vi "Lengmure_s_probe2.vi"() -> ()   [LabVIEW 2013]
uses:
  <vilib>/Instr/_visa.llb/VISA Configure Serial Port (Instr).vi
  <vilib>/Utility/file.llb/Write To Spreadsheet File (DBL).vi
  convert.dll
panel:
  out "?":dynamicdata(graph)
  in  "Tab Control":T1(tab)
  in  "Start":bool
  out "Имя соединения":refnum<visa-resource-name>
  in  "Компорт":refnum<visa-resource-name>="COM4"
  in  "Скорость передачи":u32=9600
  in  "Токоограничитель":bool=TRUE
  in  "50 герцовый фильтр":bool
  in  "Опорное напряжение АЦП, Вольты":dbl=5.0
  in  "Разрядность АЦП":u8=10
  in  "Реле 4":bool
  in  "Реле 3":bool
  in  "Реле 2":bool
  in  "Реле 1":bool
  in  "Go":bool
  in  "Save":bool
  in  "Clear":bool
  in  "stop":bool
  out "U-I Diagram":cluster{dbl[], dbl[]}(graph)
  in  "Команда":string
  out "Отправка команд /Чтение данных":bool
  in  "Начальное напряжение(0..255)":u8
  in  "Диапазон напряжения(0..255)":u8=255
  in  "Задержка (10 мс)(0..255)":u8=1
  in  "Количество шагов(0..255)":u8=255
  in  "Повторы(0..255)":u8=1
  in  "Время паузы данных(мс)":u32=1000
  in  "Обратный коэффицент делителя напряжения, Безразм":dbl=49.0
  in  "Сопротивление шунта, Ом":dbl=22.0
  out "Время выполнения операции(мсек)":u32
  out "Передача команд":errorcluster
  out "Инициализация":errorcluster
  out "Модуль считывания данных":errorcluster
  out "Закрытие соединения":errorcluster
  out "Вспомогательная переменная времени начала команды":u32
  out "Вспомогательная переменная времени последних принятых данных":u32
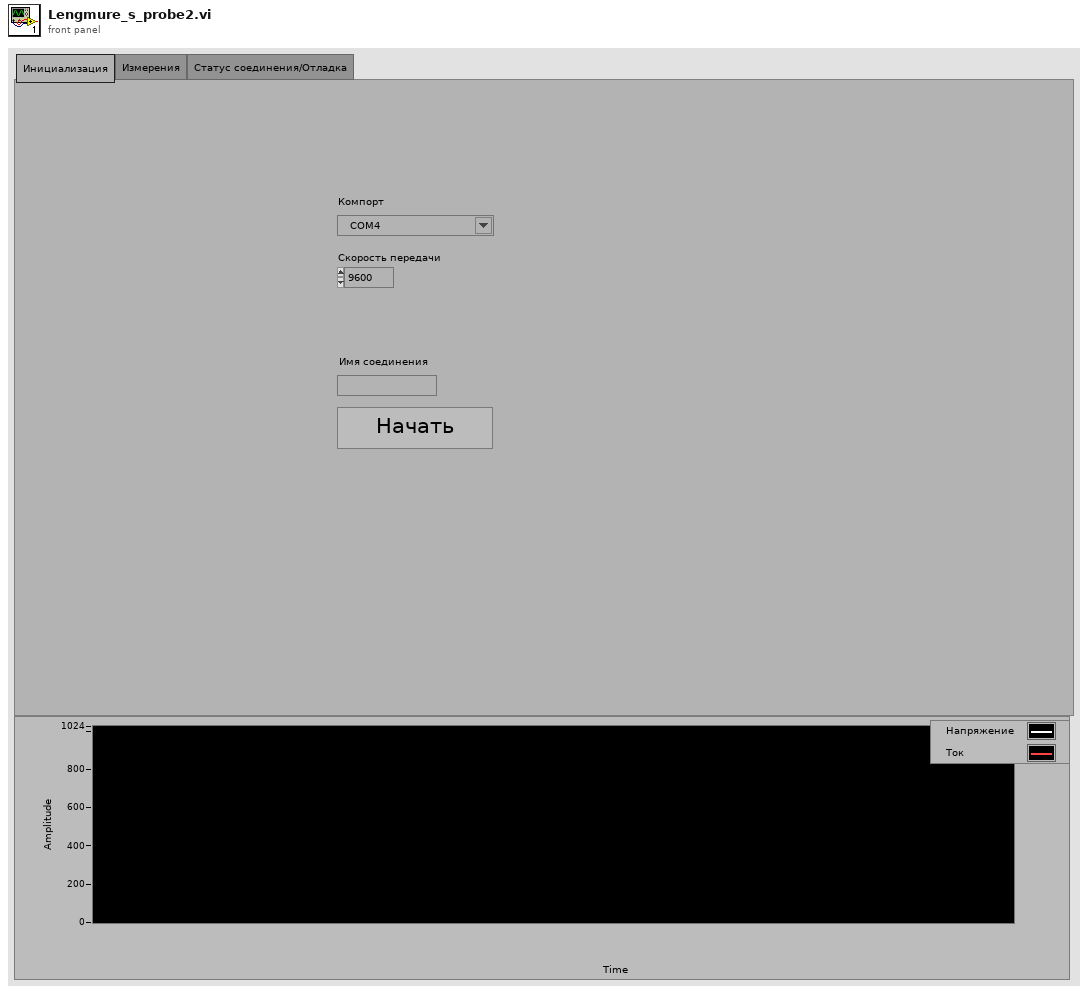
[diagram p1: front panel]
types:
  T1 = enum32{"Инициализация", "Измерения", "Статус соединения/Отладка"}
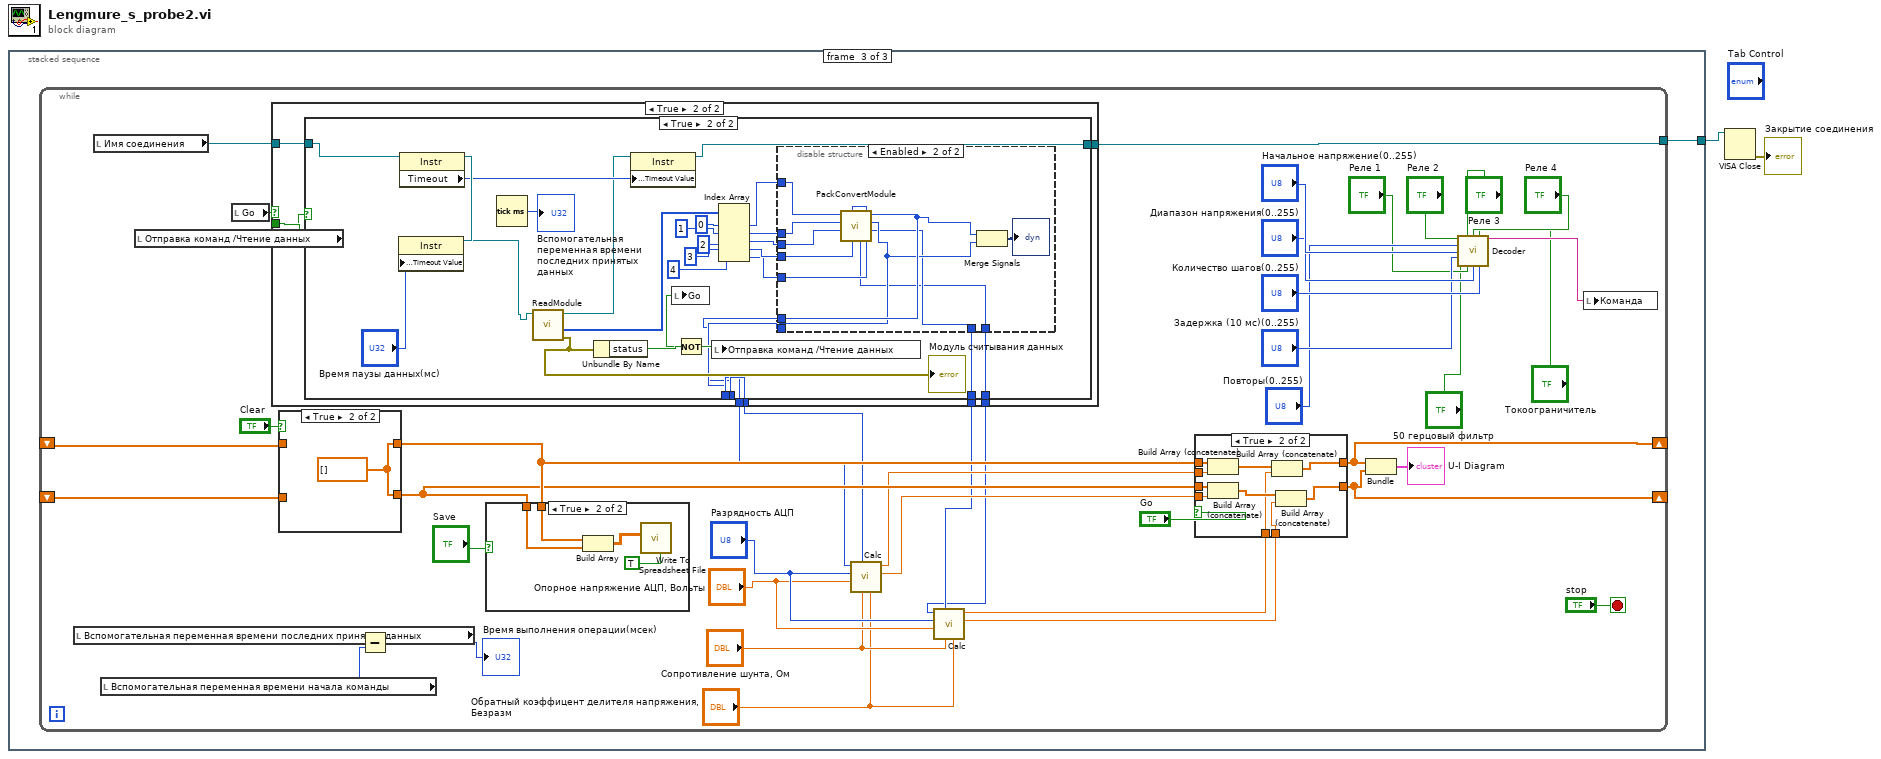
[diagram p0: block diagram]
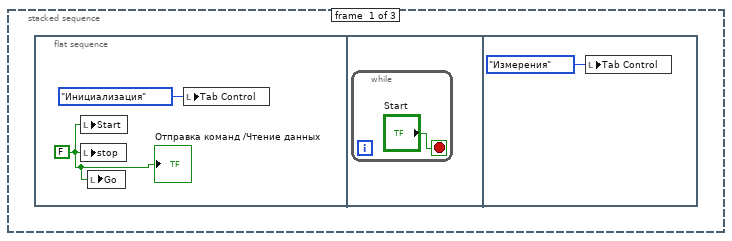
[diagram p2: hidden frame]
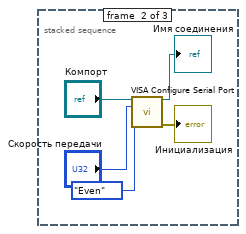
[diagram p3: hidden frame]
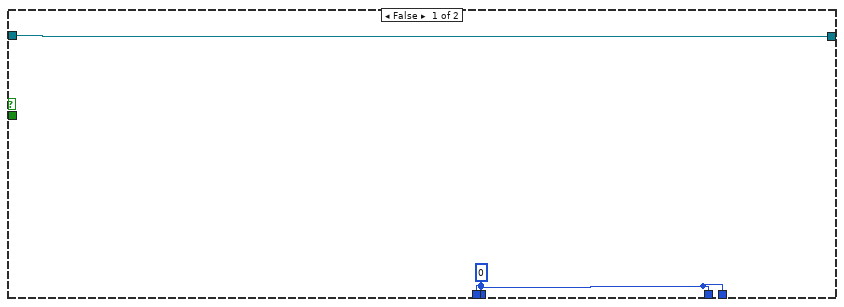
[diagram p4: hidden frame]
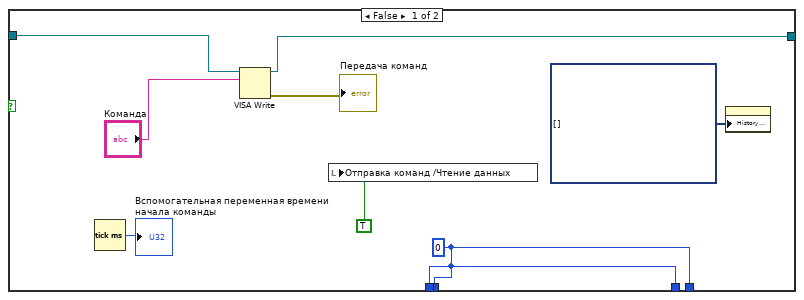
[diagram p5: hidden frame]
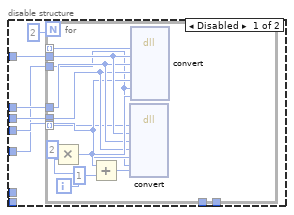
[diagram p6: hidden frame]
diagram:
  n1 = stacked-sequence {
    tunnel: [_ _ w12] -> w2
    frame #0 {
      n2 = flat-sequence {
        frame #0 {
          w3 = FALSE ("Start")
          n3 = local write "Start"(w3) -> ()
          n4 = local write "stop"(w3) -> ()
          n5 = local write "Go"(w3) -> ()
          n6 = local write "Tab Control"(enum32{"Инициализация", "Измерения"}."Инициализация" ("Tab Control")) -> ()
          "Отправка команд /Чтение данных" <- w3
        }
        frame #1 {
          n7 = while {
            stop <- "Start" stop-if-true
          }
        }
        frame #2 {
          n8 = local write "Tab Control"(enum32{"Инициализация", "Измерения"}."Измерения" ("Tab Control")) -> ()
        }
      }
    }
    frame #1 {
      n9 = call-poly "VISA Configure Serial Port"("VISA resource name"="Компорт", "baud rate (9600)"="Скорость передачи", "parity (0:none)"=enum16{"None", "Odd", "Even", "Mark", "Space"}."Even") -> ("VISA resource name out"=→"Имя соединения":refnum<visa-resource-name>, "error out"=→"Инициализация":errorcluster)  [unwired: 11 in]
    }
    frame #2 {
      n10 = while {
        shift-right: [w41] -> _
        shift-left: _ -> [w53]
        shift-right: [w40] -> _
        shift-left: _ -> [w52]
        tunnel: [w45] -> w12
        stop <- "stop" stop-if-true
        n11 = local read "Вспомогательная переменная времени последних принятых данных"() -> (w22:u32)
        n12 = local read "Имя соединения"() -> (w46:refnum<visa-resource-name>)
        n13 = local read "Вспомогательная переменная времени начала команды"() -> (w23:u32)
        n14 = local read "Отправка команд /Чтение данных"() -> (w43:bool)
        n15 = local read "Go"() -> (w44:bool)
        n16 = case shown="True" w44 {
          tunnel: [w55 w63] -> w27
          tunnel: [w55 w62] -> w26
          tunnel: w46 -> [w56 w61]
          tunnel: [w56 w60] -> w45
          tunnel: w43 -> [_ w59]
          tunnel: [w55 w58] -> w20
          tunnel: [w55 w57] -> w19
          frame False {
            w55 = u16 0 ("return type")
          }
          frame True {
            n17 = case shown="True" w59 {
              tunnel: [w64 w75] -> w63
              tunnel: [w64 w76] -> w62
              tunnel: w61 -> [w71 w93]
              tunnel: [w70 w92] -> w60
              tunnel: [w64 w73] -> w58
              tunnel: [w64 w72] -> w57
              frame False {
                w64 = 0
                n18 = Tick Count (ms)() -> (millisecond timer value=→"Вспомогательная переменная времени начала команды":u32)
                n19 = VISA Write(VISA resource name=w71, write buffer="Команда") -> (VISA resource name out=w70:refnum<visa-resource-name>, error out=→"Передача команд":errorcluster)  [unwired: 1 in, 1 out]
                n20 = local write "Отправка команд /Чтение данных"(TRUE) -> ()
                n21 = property class="WFChart (strict)"("History Data"=dynamicdata[] []) -> ()  [unwired: 2 in, 2 out]
              }
              frame True {
                n22 = property class="Instr"(reference=w93) -> (reference out=w94:refnum<visa-resource-name>, "Timeout"=w91:u32)  [unwired: 1 in, 1 out]
                n23 = property class="Instr"(reference=w94, "General Settings:Timeout Value"="Время паузы данных(мс)") -> (reference out=w80:refnum<visa-resource-name>)  [unwired: 1 in, 1 out]
                n24 = Tick Count (ms)() -> (millisecond timer value=→"Вспомогательная переменная времени последних принятых данных":u32)
                n25 = call "ReadModule.vi"("VISA Refnum in"=w80) -> ("error out"=w77:errorcluster, "unsigned byte array"=w78:u8[], "VISA Refnum out"=w79:refnum<visa-resource-name>)  [unwired: 7 in, 1 out]
                "Модуль считывания данных" <- w77
                n26 = Unbundle By Name(w77) -> ("status"=w90:bool)
                n27 = property class="Instr"(reference=w79, "General Settings:Timeout Value"=w91) -> (reference out=w92:refnum<visa-resource-name>)  [unwired: 1 in, 1 out]
                n28 = Not(x=w90) -> (.not. x?=w89:bool)
                n29 = local write "Go"(w89) -> ()
                n30 = local write "Отправка команд /Чтение данных"(w89) -> ()
                n31 = Index Array(array=w78, index #1=0 ("index"), index #2=1 ("index"), index #3=2 ("index"), index #4=3 ("index"), index #5=4 ("index")) -> (element #1=w85:u8, element #2=w84:u8, element #3=w83:u8, element #4=w82:u8, element #5=w81:u8)
                n32 = disable-structure shown="Enabled" {
                  disable-tunnel: w85 -> [w102 w124]
                  disable-tunnel: w84 -> [w101 w123]
                  disable-tunnel: w83 -> [w100 w122]
                  disable-tunnel: w82 -> [w99 w121]
                  disable-tunnel: w81 -> [w98 w120]
                  disable-tunnel: [_ w118] -> w76
                  disable-tunnel: [_ w119] -> w75
                  disable-tunnel: [_ w117] -> w73
                  disable-tunnel: [_ w116] -> w72
                  frame Disabled {
                    n33 = for {
                      N: 2 -> [_]
                      tunnel: w102 -> [w110]
                      tunnel: w101 -> [w109]
                      tunnel: w100 -> [w108]
                      tunnel: w99 -> [w107]
                      tunnel: w98 -> [w106]
                      tunnel: [w105] -> _ mode=indexing
                      tunnel: [w104] -> _ mode=indexing
                      i -> [w115]
                      n34 = Multiply(x=2, y=w115) -> (x*y=w113:i32)
                      n35 = Add(x=w113, y=1) -> (x+y=w111:i32)
                      n36 = dll-call lib="PTH1ђabs CUsers\nР”РµРЅРёСЃDesktopProjectSpaceР Р°Р·СЂР°Р±РѕС‚РєР°Lengmure's probeArduino Duemilianove(ATmega328)Labviewconvert.dll" fn="convert"("a0"=w110, "a1"=w109, "a2"=w108, "a3"=w107, "a4"=w106, "param"=w111) -> ("return type"=w104:u16)  [unwired: 9 in, 2 out]
                      n37 = dll-call lib="PTH1ђabs CUsers\nР”РµРЅРёСЃDesktopProjectSpaceР Р°Р·СЂР°Р±РѕС‚РєР°Lengmure's probeArduino Duemilianove(ATmega328)Labviewconvert.dll" fn="convert"("a0"=w110, "a1"=w109, "a2"=w108, "a3"=w107, "a4"=w106, "param"=w113) -> ("return type"=w105:u16)  [unwired: 9 in, 2 out]
                    }
                  }
                  frame Enabled {
                    n38 = call "PackConvertModule.vi"("3 in"=w121, "4"=w120, "2 in"=w122, "1 in"=w123, "0 in"=w124) -> ("2 out"=w117:u16, "1 out"=w118:u16, "0 out"=w119:u16, "3 out"=w116:u16)  [unwired: 3 in]
                    n39 = Merge Signals(w119, w118) -> (→"?":dynamicdata)
                  }
                }
              }
            }
          }
        }
        n40 = case shown="True" "Clear" {
          tunnel: w53 -> [w143 _]
          tunnel: w52 -> [w142 _]
          tunnel: [w143 w144] -> w48
          tunnel: [w142 w144] -> w47
          frame False {
          }
          frame True {
            w144 = dbl[] []
          }
        }
        n41 = Subtract(x=w22, y=w23) -> (x-y=→"Время выполнения операции(мсек)":u32)
        n42 = case shown="True" "Save" {
          tunnel: w48 -> [_ w141]
          tunnel: w47 -> [_ w140]
          frame False {
          }
          frame True {
            n43 = Build Array(w141, w140) -> (w139:dbl[][])
            n44 = call-poly <vilib>:"Write To Spreadsheet File.vi"("transpose? (no:F)"=TRUE, "2D data"=w139) -> ()  [unwired: 6 in, 1 out]
          }
        }
        n45 = call "Calc.vi"("Обратный коэффицент делителя напряжения, Безразм"="Обратный коэффицент делителя напряжения, Безразм", "Сопротивление шунта, Ом"="Сопротивление шунта, Ом", "0 in"=w27, "Опорное напряжение АЦП, Вольты"="Опорное напряжение АЦП, Вольты", "Разрядность АЦП"="Разрядность АЦП", "1 in"=w26) -> ("Numeric 2"=w29:dbl, "Numeric"=w28:dbl)  [unwired: 4 in]
        n46 = call "Calc.vi"("Обратный коэффицент делителя напряжения, Безразм"="Обратный коэффицент делителя напряжения, Безразм", "Сопротивление шунта, Ом"="Сопротивление шунта, Ом", "0 in"=w20, "Опорное напряжение АЦП, Вольты"="Опорное напряжение АЦП, Вольты", "Разрядность АЦП"="Разрядность АЦП", "1 in"=w19) -> ("Numeric 2"=w13:dbl, "Numeric"=w14:dbl)  [unwired: 4 in]
        n47 = case shown="True" "Go" {
          tunnel: w48 -> [w126 w137]
          tunnel: w47 -> [w127 w136]
          tunnel: [w126 w133] -> w41
          tunnel: [w127 w132] -> w40
          tunnel: w29 -> [_ w134]
          tunnel: w28 -> [_ w135]
          tunnel: w14 -> [_ w129]
          tunnel: w13 -> [_ w128]
          frame False {
          }
          frame True {
            n48 = Build Array (concatenate)(w137, w135) -> (w131:dbl[])
            n49 = Build Array (concatenate)(w136, w134) -> (w130:dbl[])
            n50 = Build Array (concatenate)(w131, w129) -> (w133:dbl[])
            n51 = Build Array (concatenate)(w130, w128) -> (w132:dbl[])
          }
        }
        n52 = Bundle(w41, w40) -> (→"U-I Diagram":cluster{dbl[], dbl[]})  [unwired: 1 in]
        n53 = call "Decoder.vi"("Реле in"="Реле 2", "Реле 3"="Реле 3", "Реле 4"="Реле 4", "Токоограничитель"="Токоограничитель", "Повторы(0..255)"="Повторы(0..255)", "Начальное напряжение(0..255)"="Начальное напряжение(0..255)", "Задержка (10 мс)(0..255)"="Задержка (10 мс)(0..255)", "50 герцовый фильтр"="50 герцовый фильтр", "Реле 1"="Реле 1", "Диапазон напряжения(0..255)"="Диапазон напряжения(0..255)", "Количество шагов(0..255)"="Количество шагов(0..255)") -> ("string"=w30:string)  [unwired: 4 in]
        n54 = local write "Команда"(w30) -> ()
      }
    }
  }
  n55 = VISA Close(VISA resource name=w2) -> (error out=→"Закрытие соединения":errorcluster)  [unwired: 1 in]
